vi "Scale-Rotate.vi"(4 "offset Y":dbl format="%0.2f", 5 "Rotation (deg)":dbl, 6 "offset X":dbl format="%0.2f", 7 "Scale":dbl=5.0, 9 "Scale by":enum16{"X", "Y", "XY"}(ring)=enum."Y", 10 "Y in":ext[](array[numeric]), 11 "X in":ext[](array[numeric])) -> (2 "Y out":dbl[](array[numeric]), 3 "X out":dbl[](array[numeric]))   [LabVIEW 2014]
doc: "André Romero - 2016\nandretec@ifsc.usp.br\n\nRotate, Scale coordenates\nOffset XY"
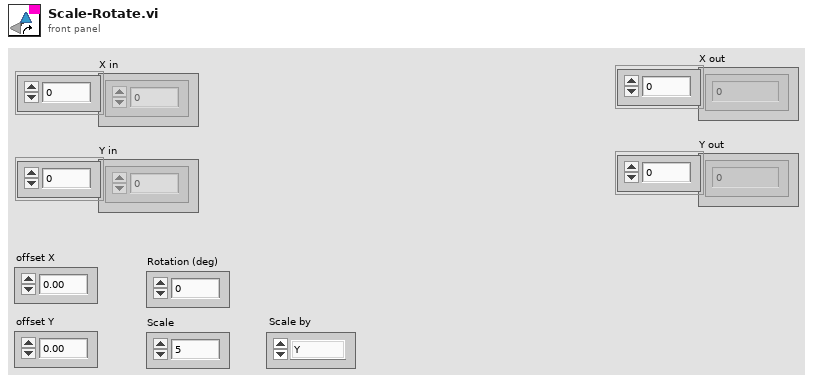
[diagram p1: front panel]
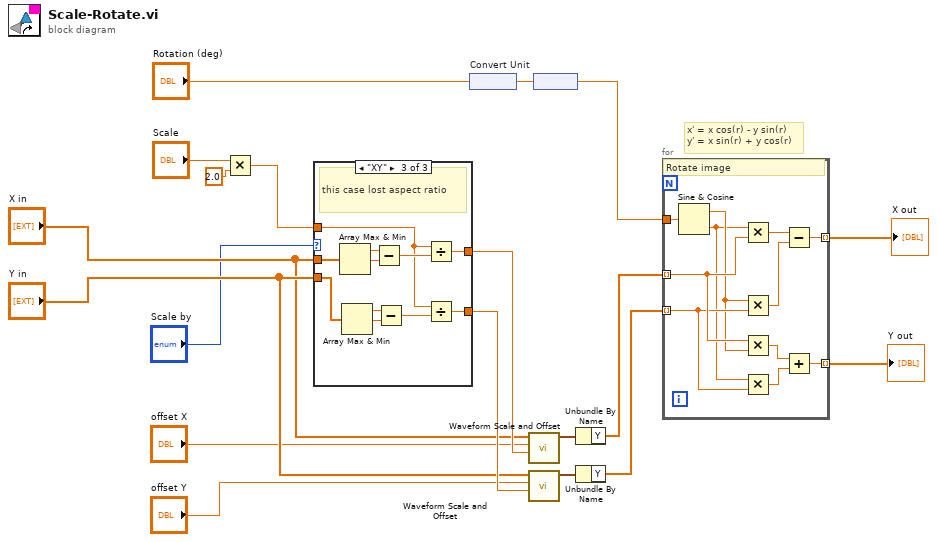
[diagram p0: block diagram]
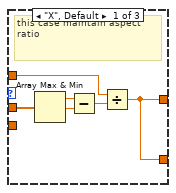
[diagram p2: hidden frame]
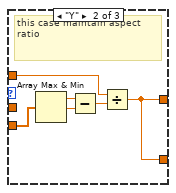
[diagram p3: hidden frame]
diagram:
  # "x' = x cos(r) - y sin(r)\ny' = x sin(r) + y cos(r)"
  n1 = Multiply(x="Scale", y=2.0) -> (x*y=w4:dbl)
  n2 = case shown="\"XY\"" "Scale by" {
    tunnel: "X in" -> [w25 _ w42]
    tunnel: [w20 w26 w38] -> w19
    tunnel: w4 -> [w21 w28 w33]
    tunnel: "Y in" -> [_ w27 w34]
    tunnel: [w20 w26 w32] -> w18
    frame "X", Default {
      # "this case maintain aspect ratio"
      n3 = Array Max & Min(array=w25) -> (max value=w24:ext, min value=w23:ext)  [unwired: 2 out]
      n4 = Subtract(x=w24, y=w23) -> (x-y=w22:ext)
      n5 = Divide(x=w21, y=w22) -> (x/y=w20:ext)
    }
    frame "Y" {
      # "this case maintain aspect ratio"
      n6 = Array Max & Min(array=w27) -> (max value=w31:ext, min value=w30:ext)  [unwired: 2 out]
      n7 = Subtract(x=w31, y=w30) -> (x-y=w29:ext)
      n8 = Divide(x=w28, y=w29) -> (x/y=w26:ext)
    }
    frame "XY" {
      # "this case lost aspect ratio"
      n9 = Array Max & Min(array=w42) -> (max value=w41:ext, min value=w40:ext)  [unwired: 2 out]
      n10 = Array Max & Min(array=w34) -> (max value=w37:ext, min value=w36:ext)  [unwired: 2 out]
      n11 = Subtract(x=w41, y=w40) -> (x-y=w39:ext)
      n12 = Subtract(x=w37, y=w36) -> (x-y=w35:ext)
      n13 = Divide(x=w33, y=w39) -> (x/y=w38:ext)
      n14 = Divide(x=w33, y=w35) -> (x/y=w32:ext)
    }
  }
  n15 = node "Convert Unit"("Rotation (deg)") -> (w16:dbl[unit])
  n16 = call <vilib>:"Waveform Scale and Offset.vi"("scale"=w19, "offset"="offset X", "waveform in"="X in") -> ("waveform out"=w7:waveform(dbl))  [unwired: 7 in, 1 out]
  n17 = call <vilib>:"Waveform Scale and Offset.vi"("scale"=w18, "offset"="offset Y", "waveform in"="Y in") -> ("waveform out"=w8:waveform(dbl))  [unwired: 7 in, 1 out]
  n18 = node(w16) -> (w17:dbl)
  n19 = Unbundle By Name(w7) -> ("Y"=w11:dbl[])
  n20 = Unbundle By Name(w8) -> ("Y"=w12:dbl[])
  n21 = for {
    tunnel: w11 -> [w49] mode=indexing
    tunnel: w12 -> [w48] mode=indexing
    tunnel: w17 -> [w53]
    tunnel: [w50] -> w13 mode=indexing
    tunnel: [w44] -> w14 mode=indexing
    # "Rotate image"
    n22 = Sine & Cosine(0:w53) -> (1:w47:dbl, 2:w43:dbl)
    n23 = Multiply(x=w43, y=w49) -> (x*y=w52:dbl)
    n24 = Multiply(x=w47, y=w48) -> (x*y=w51:dbl)
    n25 = Multiply(x=w49, y=w47) -> (x*y=w46:dbl)
    n26 = Multiply(x=w43, y=w48) -> (x*y=w45:dbl)
    n27 = Subtract(x=w52, y=w51) -> (x-y=w50:dbl)
    n28 = Add(x=w46, y=w45) -> (x+y=w44:dbl)
  }
  "Y out" <- w14
  "X out" <- w13
